vi "practica3.vi"() -> ()   [LabVIEW 2021]
uses:
  <vilib>/ptbypt/NI_PtbyPt.lvlib
panel:
  out "Comparacion de señales":T1(graph)
  in  "stop":bool
  in  "Tf":dbl
  in  "Ts":dbl
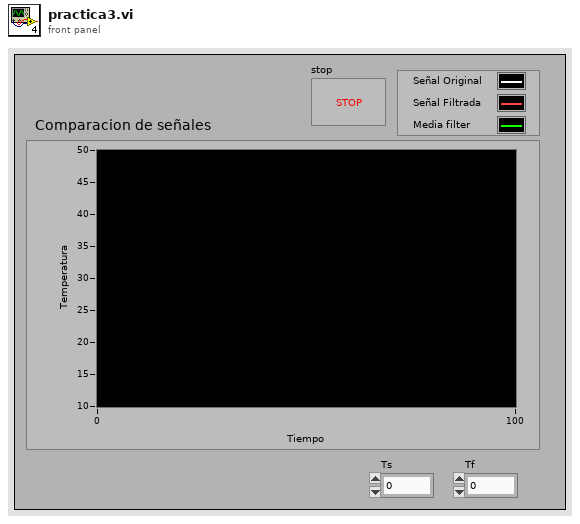
[diagram p1: front panel]
types:
  T1 = cluster{dbl, "señal filtrada":dbl, "Filtered x":dbl}
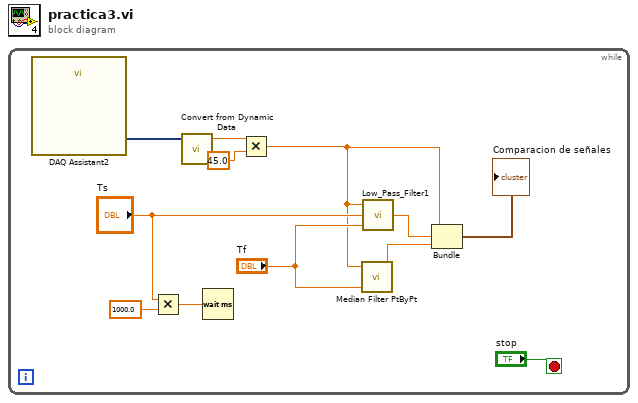
[diagram p0: block diagram]
diagram:
  n1 = while {
    stop <- "stop" stop-if-true
    n2 = call "DAQ Assistant2"() -> ("data"=w3:dynamicdata)  [unwired: 17 in, 2 out]
    n3 = Multiply(x="Ts", y=1000.0) -> (x*y=w10:dbl)
    n4 = call "Convert from Dynamic Data"("Dynamic Data Type"=w3) -> ("Scalar"=w9:dbl)  [unwired: 3 in]
    n5 = Wait (ms)(milliseconds to wait=w10) -> ()  [unwired: 1 out]
    n6 = Multiply(x=w9, y=45.0) -> (x*y=w1:dbl)
    n7 = call <vilib>:"Median Filter PtByPt.vi"("rank"="Tf", "x"=w1) -> ("Filtered x"=w5:dbl)  [unwired: 2 in, 1 out]
    n8 = call "Low_Pass_Filter1.vi"("Tf"="Tf", "Ts"="Ts", "yk"=w1) -> ("señal filtrada"=w4:dbl)
    n9 = Bundle(w1, "señal filtrada"=w4, "Filtered x"=w5) -> (→"Comparacion de señales":T1)  [unwired: 1 in]
  }
